vi "Setup subWorker - gRPC Client.vi"(8 "error in":errorcluster, 11 "gRPC Client Tester in":refnum<class "gRPC Client Tester.lvclass">) -> (0 "error out":errorcluster, 3 "gRPC Client Tester out":refnum<class "gRPC Client Tester.lvclass">)   [LabVIEW 2019, in "gRPC Client Tester.lvclass"]
doc: "This VI sets up the framework parameters of a statically-linked subWorker."
uses:
  gRPC Client Tester.lvclass
  gRPC Client/gRPC Client/gRPC Client.lvclass
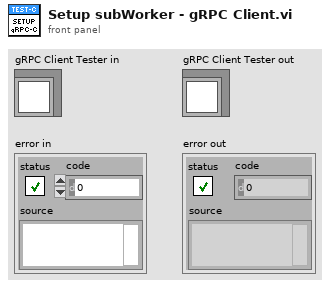
[diagram p1: front panel]
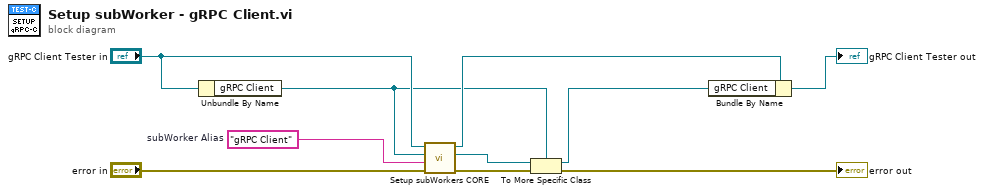
[diagram p0: block diagram]
diagram:
  w6 = "gRPC Client"  # subWorker Alias
  n1 = Unbundle By Name("gRPC Client Tester in") -> ("gRPC Client"=w3:refnum<class "gRPC Client.lvclass">)
  n2 = call-dynamic "Setup subWorkers CORE.vi"("error in"="error in", "subWorker Alias"=w6, "subWorker"=w3, "Worker"="gRPC Client Tester in") -> ("error out"=w5:errorcluster, "subWorker out"=w1:refnum<class "Worker.lvclass">, "Worker out"=w8:refnum<class "gRPC Client Tester.lvclass">)  [unwired: 5 in]
  n3 = To More Specific Class(target class=w3, reference=w1, error in=w5) -> (specific class reference=w2:refnum<class "gRPC Client.lvclass">, error out=→"error out":errorcluster)
  n4 = Bundle By Name(cluster=w8, "gRPC Client"=w2) -> (→"gRPC Client Tester out":refnum<class "gRPC Client Tester.lvclass">)
